vi "m100RecipeToExcel.vi"() -> ()   [LabVIEW 2012]
uses:
  <vilib>/addons/database/Auxilliary.llb/DB Tools Cursor Type.ctl
  <vilib>/Utility/NIReport.llb/NI_report.lvclass
  <vilib>/addons/database/Connection.llb/DB Tools Open Connec (Path).vi
  <vilib>/addons/database/Connection.llb/Conn Execute.vi
  <vilib>/addons/database/Recordset.llb/Rec Fetch Recordset Data (R).vi
  <vilib>/addons/database/Recordset.llb/Rec Destroy - Connection.vi
  <vilib>/addons/database/_DB Variant To Data/Database Variant To Data.xnode
  <vilib>/Utility/NIReport.llb/Excel/NI_Excel.lvclass
  <vilib>/addons/database/NI_Database_API.lvlib
panel:
  in  "?":cluster{"start row":i32, "start column":i32}
  out "recordset data":variant[][](array[variant])
  out "error out 4":errorcluster
  out "error out":errorcluster
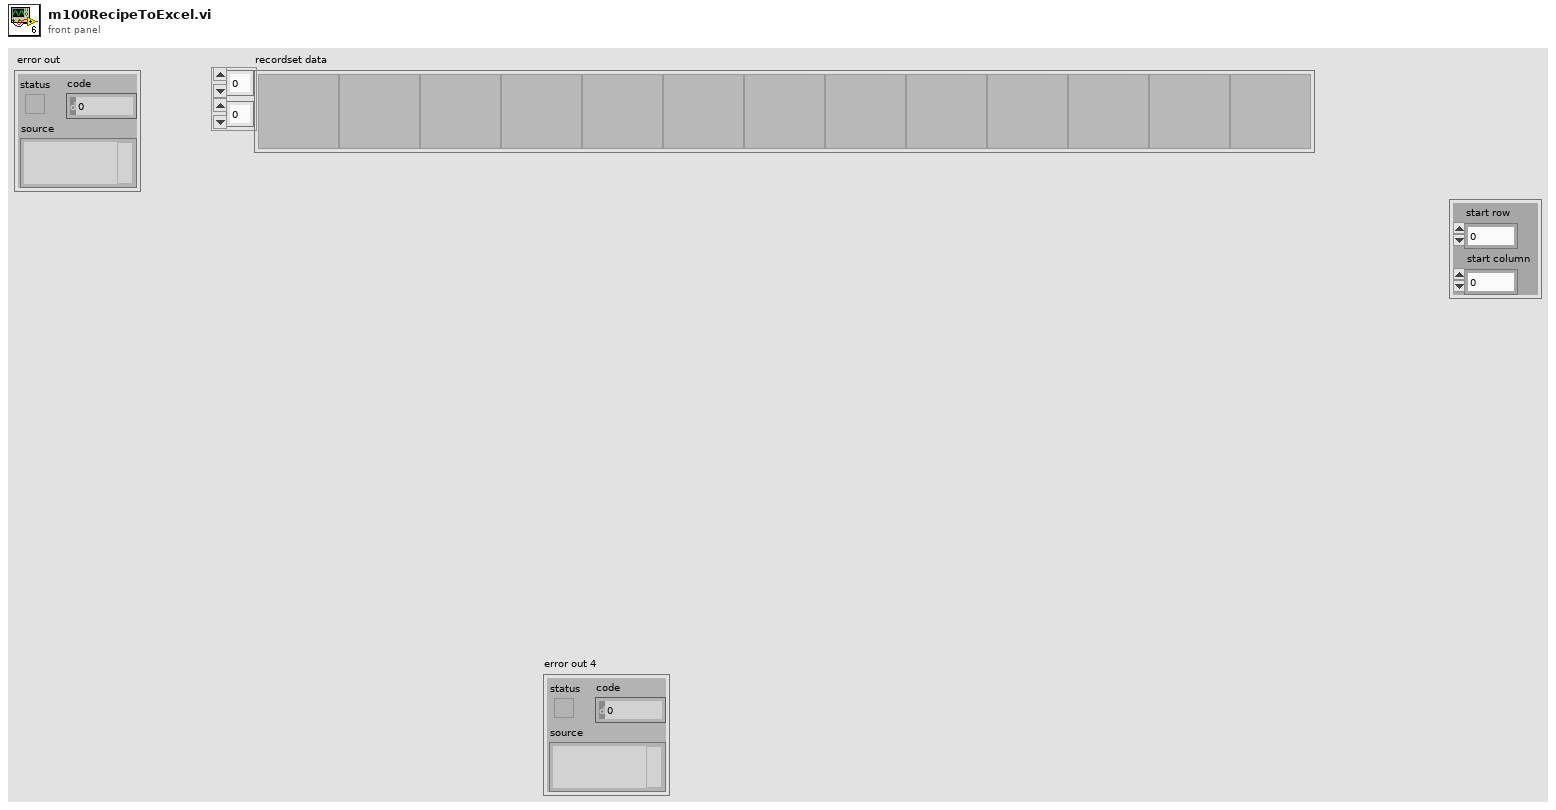
[diagram p1: front panel]
types:
  T1 = enum16{"Standard Report", "HTML", "Word", "Excel"}
  T2 = typedef "NI_Database_API.lvlib/DB Tools Cursor Type.ctl" = enum16{"forward-only", "keyset", "dynamic", "static"}
  T3 = typedef "NI_Database_API.lvlib/Conn ObjectReference.ctl" = refnum<k1>
  T4 = typedef "NI_Database_API.lvlib/Rec ObjectReference.ctl" = refnum<k1>
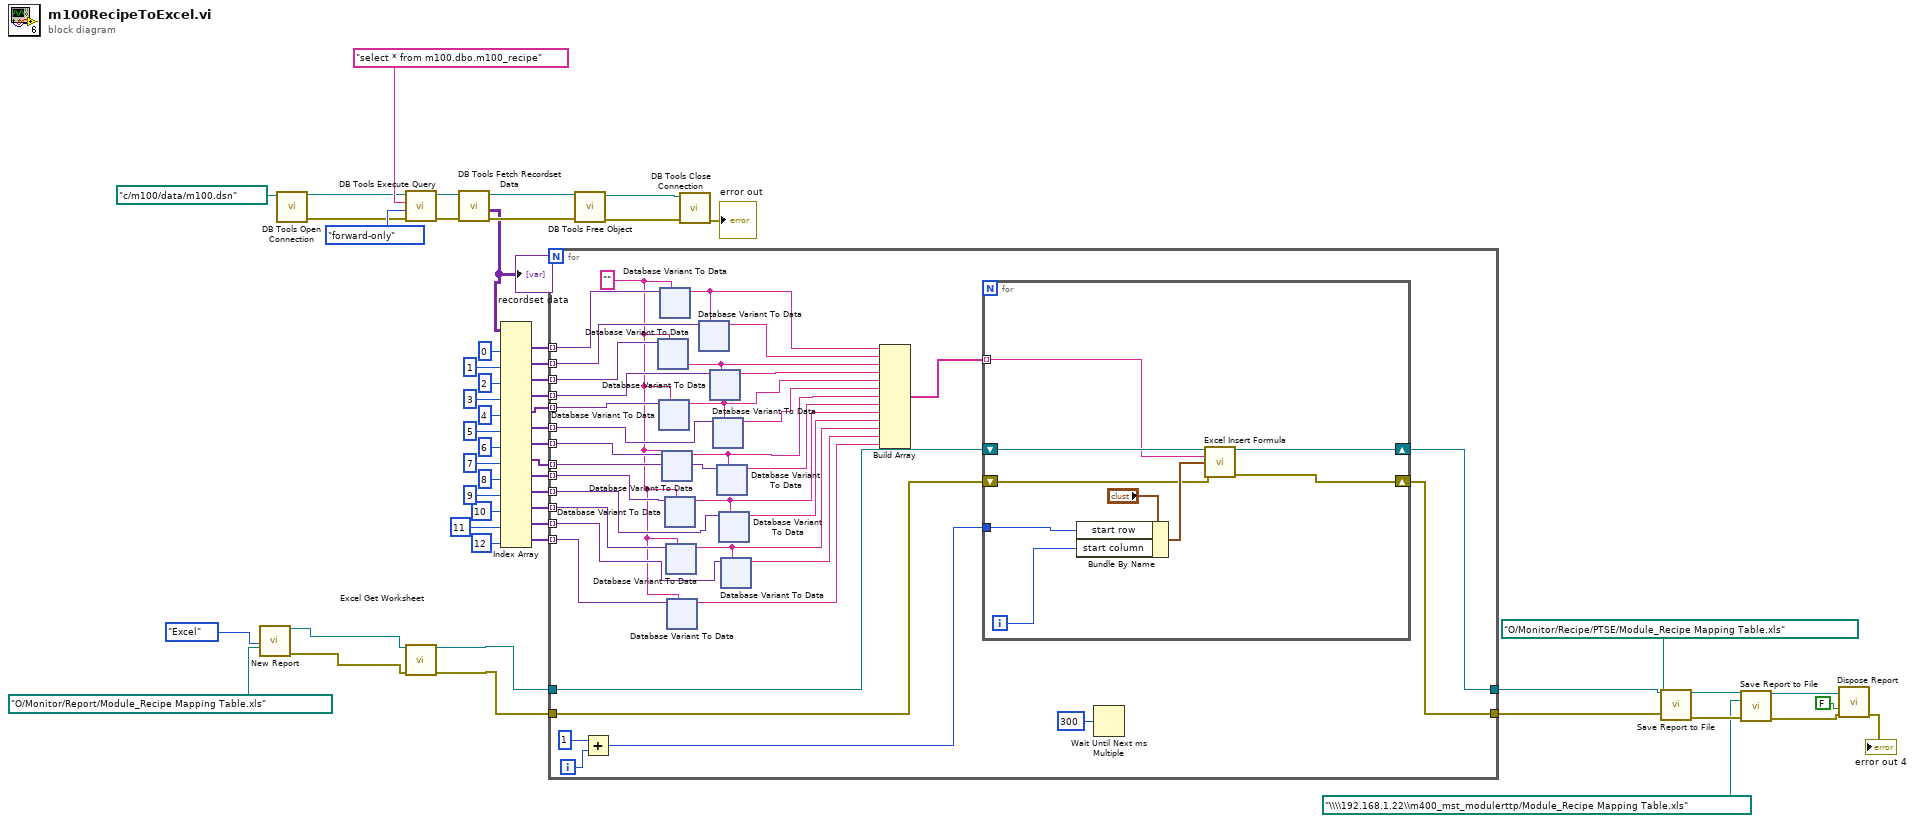
[diagram p0: block diagram]
diagram:
  n1 = call <vilib>:"New Report.vi"("report type"=T1."Excel" ("Report Type"), "template (empty)"=path "O:/Monitor/Report/Module_Recipe Mapping Table.xls") -> ("report out"=w14:refnum<class "NI_report.lvclass">, "error out"=w13:errorcluster)  [unwired: 12 in]
  n2 = call-poly <vilib>:"DB Tools Open Connection.vi"("connection information"=path "c:/m100/data/m100.dsn") -> ("error out"=w21:errorcluster, "connection reference"=w22:T3)  [unwired: 7 in]
  n3 = call-poly <vilib>:"DB Tools Execute Query.vi"("error in (no error)"=w21, "cursor type"=DB_Tools_Cursor_Type."forward-only", "SQL query"="select * from m100.dbo.m100_recipe", "connection reference"=w22) -> ("error out"=w55:errorcluster, "recordset reference"=w54:T4)  [unwired: 4 in]
  n4 = call <vilib>:"Excel Get Worksheet.vi"("report in"=w14, "error in (no error)"=w13) -> ("report out"=w25:refnum<class "NI_report.lvclass">, "error out"=w24:errorcluster)  [unwired: 12 in]
  n5 = call-poly <vilib>:"DB Tools Fetch Recordset Data.vi"("error in (no error)"=w55, "recordset reference"=w54) -> ("error out"=w52:errorcluster, "recordset data"=w50:variant[][], "recordset reference out"=w53:T4)  [unwired: 3 in]
  "recordset data" <- w50
  n6 = Index Array(array=w50, index (col) #1=0 ("disabled index (col)"), index (col) #2=1 ("index (col)"), index (col) #3=2 ("index (col)"), index (col) #4=3 ("index (col)"), index (col) #5=4 ("index (col)"), index (col) #6=5 ("index (col)"), index (col) #7=6 ("index (col)"), index (col) #8=7 ("index (col)"), index (col) #9=8 ("index (col)"), index (col) #10=9 ("index (col)"), index (col) #11=10 ("index (col)"), index (col) #12=11 ("index (col)"), index (col) #13=12 ("index (col)")) -> (element #1=w47:variant[], element #2=w46:variant[], element #3=w45:variant[], element #4=w34:variant[], element #5=w33:variant[], element #6=w32:variant[], element #7=w31:variant[], element #8=w30:variant[], element #9=w29:variant[], element #10=w28:variant[], element #11=w27:variant[], element #12=w26:variant[], element #13=w1:variant[])  [unwired: 13 in]
  n7 = for {
    tunnel: w47 -> [w91] mode=indexing
    tunnel: w46 -> [w90] mode=indexing
    tunnel: w45 -> [w89] mode=indexing
    tunnel: w34 -> [w87] mode=indexing
    tunnel: w33 -> [w83] mode=indexing
    tunnel: w32 -> [w81] mode=indexing
    tunnel: w31 -> [w79] mode=indexing
    tunnel: w30 -> [w76] mode=indexing
    tunnel: w29 -> [w75] mode=indexing
    tunnel: w28 -> [w74] mode=indexing
    tunnel: w27 -> [w71] mode=indexing
    tunnel: w26 -> [w70] mode=indexing
    tunnel: w25 -> [w62]
    tunnel: w24 -> [w61]
    tunnel: [w64] -> w10
    tunnel: [w63] -> w9
    tunnel: w1 -> [w58] mode=indexing
    i -> [w67]
    w59 = ""
    n8 = Add(x=1, y=w67) -> (x+y=w60:i32)
    n9 = xnode "Database Variant To Data"("database variant"=w89, "type"=w59) -> ("data"=w85:string)  [unwired: 1 in, 1 out]
    n10 = xnode "Database Variant To Data"("database variant"=w83, "type"=w59) -> ("data"=w82:string)  [unwired: 1 in, 1 out]
    n11 = xnode "Database Variant To Data"("database variant"=w91, "type"=w59) -> ("data"=w86:string)  [unwired: 1 in, 1 out]
    n12 = xnode "Database Variant To Data"("database variant"=w79, "type"=w59) -> ("data"=w78:string)  [unwired: 1 in, 1 out]
    n13 = xnode "Database Variant To Data"("database variant"=w75, "type"=w59) -> ("data"=w73:string)  [unwired: 1 in, 1 out]
    n14 = xnode "Database Variant To Data"("database variant"=w71, "type"=w59) -> ("data"=w69:string)  [unwired: 1 in, 1 out]
    n15 = xnode "Database Variant To Data"("database variant"=w58, "type"=w59) -> ("data"=w57:string)  [unwired: 1 in, 1 out]
    n16 = xnode "Database Variant To Data"("database variant"=w90, "type"=w86) -> ("data"=w88:string)  [unwired: 1 in, 1 out]
    n17 = xnode "Database Variant To Data"("database variant"=w87, "type"=w85) -> ("data"=w84:string)  [unwired: 1 in, 1 out]
    n18 = xnode "Database Variant To Data"("database variant"=w81, "type"=w82) -> ("data"=w80:string)  [unwired: 1 in, 1 out]
    n19 = xnode "Database Variant To Data"("database variant"=w76, "type"=w78) -> ("data"=w77:string)  [unwired: 1 in, 1 out]
    n20 = xnode "Database Variant To Data"("database variant"=w74, "type"=w73) -> ("data"=w72:string)  [unwired: 1 in, 1 out]
    n21 = xnode "Database Variant To Data"("database variant"=w70, "type"=w69) -> ("data"=w68:string)  [unwired: 1 in, 1 out]
    n22 = Build Array(w86, w88, w85, w84, w82, w80, w78, w77, w73, w72, w69, w68, w57) -> (w65:string[])
    n23 = for {
      tunnel: w60 -> [w130]
      shift-right: [w128] -> w64
      shift-left: w62 -> [w126]
      shift-right: [w127] -> w63
      shift-left: w61 -> [w125]
      tunnel: w65 -> [w124] mode=indexing
      i -> [w131]
      n24 = Bundle By Name(cluster="?", "start row"=w130, "start column"=w131) -> (w129:cluster{"start row":i32, "start column":i32})
      n25 = call <vilib>:"Excel Insert Formula.vi"("report in"=w126, "formula"=w124, "start (0, 0)"=w129, "error in (no error)"=w125) -> ("report out"=w128:refnum<class "NI_report.lvclass">, "error out"=w127:errorcluster)  [unwired: 10 in]
    }
    n26 = Wait Until Next ms Multiple(millisecond multiple=u32 300) -> ()  [unwired: 1 out]
  }
  n27 = call-poly <vilib>:"DB Tools Free Object.vi"("error in (no error)"=w52, "recordset reference"=w53) -> ("error out"=w18:errorcluster, "connection reference"=w19:T3)  [unwired: 8 in]
  n28 = call <vilib>:"DB Tools Close Connection.vi"("error in (no error)"=w18, "connection reference"=w19) -> ("error out"=→"error out":errorcluster)  [unwired: 5 in]
  n29 = call-dynamic "Save Report to File.vi"("report in"=w10, "report file path"=path "O:/Monitor/Recipe/PTSE/Module_Recipe Mapping Table.xls", "error in (no error)"=w9) -> ("report out"=w7:refnum<class "NI_report.lvclass">, "error out"=w4:errorcluster)  [unwired: 11 in]
  n30 = call-dynamic "Save Report to File.vi"("report in"=w7, "report file path"=path "\\\\192.168.1.22\\m400_mst_modulerttp/Module_Recipe Mapping Table.xls", "error in (no error)"=w4) -> ("report out"=w6:refnum<class "NI_report.lvclass">, "error out"=w5:errorcluster)  [unwired: 11 in]
  n31 = call-dynamic "Dispose Report.vi"("report in"=w6, "save changes? (F)"=FALSE, "error in (no error)"=w5) -> ("error out"=→"error out 4":errorcluster)  [unwired: 12 in]
